vi "AVPP_Constructor.vi"(8 "error in (no error)":errorcluster, 10 "FAMM class":refnum<data-value>, 11 "AVPP in":refnum<class "AVPP.lvclass">) -> (0 "error out":errorcluster, 2 "AVPP_ref":refnum<data-value>, 3 "AVPP out":refnum<class "AVPP.lvclass">)   [LabVIEW 2020, in "AVPP.lvclass"]
uses:
  AVPP.lvclass
  FAMM/FAMM.lvclass
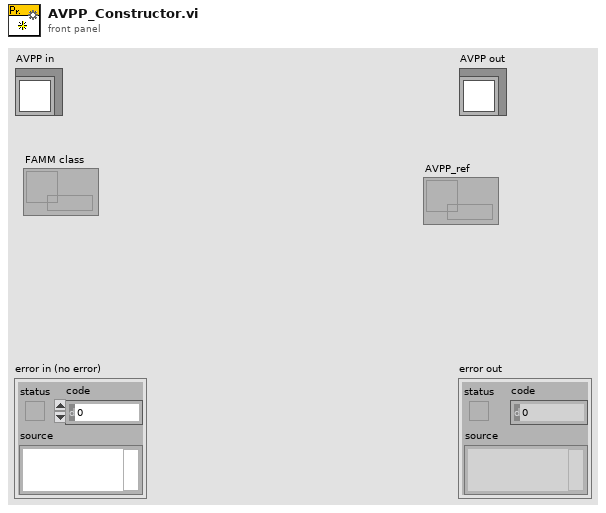
[diagram p1: front panel]
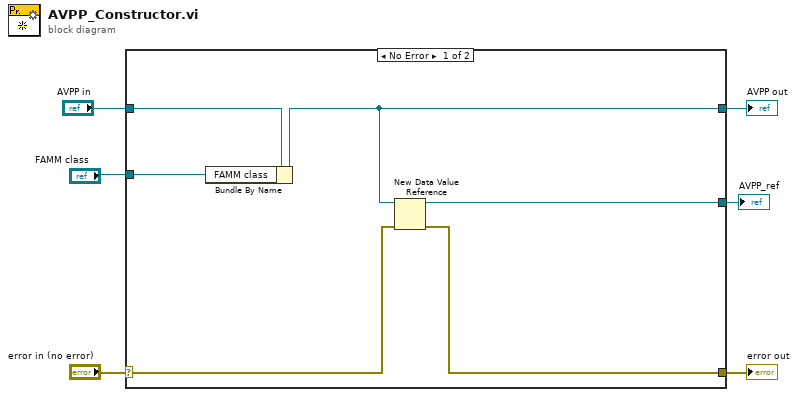
[diagram p0: block diagram]
diagram:
  n1 = case shown="No Error" "error in (no error)" {
    selector: "error in (no error)" -> [w11 w14]
    tunnel: [w10 w14] -> w5
    tunnel: [w7 w13] -> w3
    tunnel: "AVPP in" -> [w8 w13]
    tunnel: [w12 _] -> w2
    tunnel: "FAMM class" -> [w9 _]
    frame No Error {
      n2 = Bundle By Name(cluster=w8, "FAMM class"=w9) -> (w7:refnum<class "AVPP.lvclass">)
      n3 = New Data Value Reference(data value=w7, error in=w11) -> (data value reference=w12:refnum<data-value>, error out=w10:errorcluster)
    }
    frame Error {
    }
  }
  "error out" <- w5
  "AVPP out" <- w3
  "AVPP_ref" <- w2
